vi "Distances (Left, Right, Back).vi"() -> ()   [LabVIEW 2016]
uses:
  <vilib>/Analysis/baseanly.llb/Mean (DBL).vi
  <vilib>/Analysis/NI_AALBase.lvlib
panel:
  out "D: Right":dbl format="%0.2f"
  out "D: Left":dbl format="%0.2f"
  out "D: Back":dbl format="%0.2f"
  in  "Magnitude":dbl[](array[numeric])
  in  "Degrees":i32=3
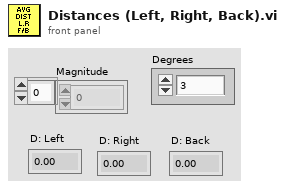
[diagram p1: front panel]
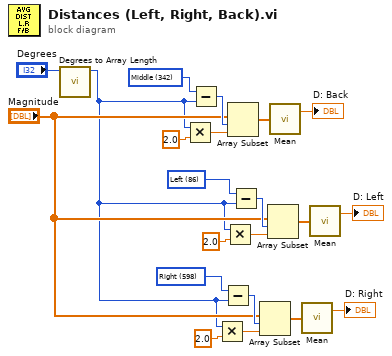
[diagram p0: block diagram]
diagram:
  w4 = u16 598 items=["Right"=598, "Left"=86, "Middle"=342]
  w10 = u16 86 items=["Right"=598, "Left"=86, "Middle"=342]
  w16 = u16 342 items=["Right"=598, "Left"=86, "Middle"=342]
  n1 = call "Degrees to Array Length.vi"("Degrees"="Degrees") -> ("Array Length"=w1:i8)  [unwired: 10 in]
  n2 = Multiply(x=w1, y=2.0) -> (x*y=w18:dbl)
  n3 = Subtract(x=w16, y=w1) -> (x-y=w20:u16)
  n4 = Multiply(x=w1, y=2.0) -> (x*y=w6:dbl)
  n5 = Subtract(x=w4, y=w1) -> (x-y=w8:u16)
  n6 = Multiply(x=w1, y=2.0) -> (x*y=w12:dbl)
  n7 = Array Subset(array="Magnitude", index=w20, length=w18) -> (w17:dbl[])
  n8 = Subtract(x=w10, y=w1) -> (x-y=w14:u16)
  n9 = Array Subset(array="Magnitude", index=w8, length=w6) -> (w5:dbl[])
  n10 = Array Subset(array="Magnitude", index=w14, length=w12) -> (w11:dbl[])
  n11 = call-poly <vilib>:"Mean.vi"("X"=w17) -> ("mean"=→"D: Back":dbl)  [unwired: 1 out]
  n12 = call-poly <vilib>:"Mean.vi"("X"=w5) -> ("mean"=→"D: Right":dbl)  [unwired: 1 out]
  n13 = call-poly <vilib>:"Mean.vi"("X"=w11) -> ("mean"=→"D: Left":dbl)  [unwired: 1 out]
